vi "Focus_KnifeEdgeFitting.vi"(3 "output control":T1, 4 "data":T2, 5 "X":dbl[](array[numeric]), 6 "a":dbl[](array[numeric])) -> (0 "error out":errorcluster, 1 "f'(X,a)":dbl[][](array[numeric]), 2 "f(X,a)":dbl[](array[numeric]))   [LabVIEW 2012]
doc: "This template is the starting point for creating a model function to be passed to the Nonlinear Curve Fit.vi."
uses:
  <vilib>/gmath/NumericalOptimization/objective function data.ctl
  <vilib>/gmath/NumericalOptimization/LM_output select.ctl
  <vilib>/gmath/NI_Gmath.lvlib
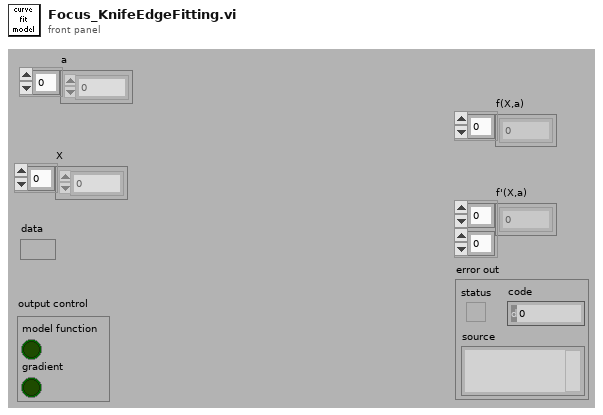
[diagram p1: front panel]
types:
  T1 = typedef "NI_Gmath.lvlib/LM_output select.ctl" = cluster{"model function":bool, "gradient":bool}
  T2 = typedef "NI_Gmath.lvlib/objective function data.ctl" = variant
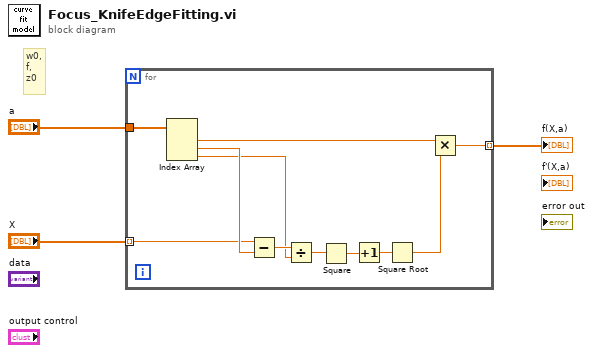
[diagram p0: block diagram]
diagram:
  # "w0,\nf,\nz0"
  n1 = for {
    tunnel: "a" -> [w14]
    tunnel: "X" -> [w12] mode=indexing
    tunnel: [w8] -> w1 mode=indexing
    n2 = Index Array(array=w14) -> (element #1=w6:dbl, element #2=w13:dbl, element #3=w7:dbl)  [unwired: 3 in]
    n3 = Subtract(x=w12, y=w13) -> (x-y=w11:dbl)
    n4 = Divide(x=w11, y=w7) -> (x/y=w10:dbl)
    n5 = Square(x=w10) -> (x^2=w5:dbl)
    n6 = Increment(x=w5) -> (x+1=w9:dbl)
    n7 = Square Root(x=w9) -> (sqrt(x)=w4:dbl)
    n8 = Multiply(x=w6, y=w4) -> (x*y=w8:dbl)
  }
  "f(X,a)" <- w1
